vi "_Read.vi"(8 "error in (no error)":errorcluster, 9 "Timeout S (0)":dbl, 10 "Bytes to Read (0)":i32, 11 "DeploySerialResource in":refnum<class "SerialResource.lvclass">) -> (0 "error out":errorcluster, 1 "Bytes Read":i32, 2 "Data":string, 3 "DeploySerialResource out":refnum<class "SerialResource.lvclass">)   [LabVIEW 2020, in "PicoG-Core.lvlib" / "SerialResource.lvclass"]
uses:
  SerialResource.lvclass
  SerialResource.lvclass/SerialResource.ctl
  <vilib>/IlluminatedG/lv-stream/stream/Stream.lvclass
  <vilib>/IlluminatedG/IG Serial Stream/Stream-Serial/Serial Client/Serial Client.lvclass
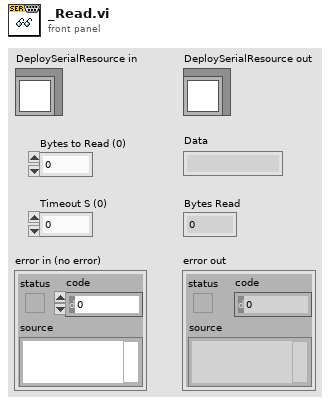
[diagram p1: front panel]
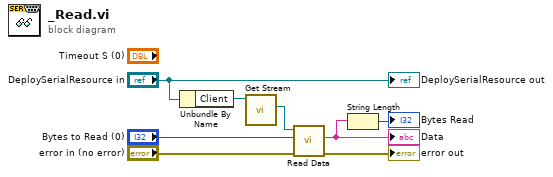
[diagram p0: block diagram]
diagram:
  n1 = Unbundle By Name("DeploySerialResource in") -> ("Client"=w7:refnum<class "Serial Client.lvclass">)
  n2 = call-dynamic "Get Stream.vi"("VISA Client in"=w7) -> ("Stream"=w6:refnum<class "Stream.lvclass">)  [unwired: 8 in, 2 out]
  n3 = call <vilib>:"Read Data.vi"("error in (no error)"="error in (no error)", "Count"="Bytes to Read (0)", "Stream in"=w6) -> ("error out"=→"error out":errorcluster, "Data"=w4:string)  [unwired: 6 in, 1 out]
  "Data" <- w4
  n4 = String Length(string=w4) -> (length=→"Bytes Read":i32)
  "DeploySerialResource out" <- "DeploySerialResource in"
